vi "MainCLEO.vi"() -> ()   [LabVIEW 2013]
uses:
  Global.vi
  <vilib>/Utility/file.llb/Write To Spreadsheet File (string).vi
panel:
  in  "stop":bool
  in  "Measured values [mm]":i32(listbox)
  out "Standard deviation":dbl min=0.0 step=0.001 format="%.2f"
  out "Mean":dbl min=0.0 step=0.001 format="%.2f"
  out "Array":dbl[][](array[numeric])
  in  "Clear":bool
  out "String 3":string
  out "String 2":string
  in  "Radio Buttons":T1(radio)
  out "Delta average":dbl format="%#.4f"
  out "Delta right":dbl format="%#.4f"
  out "Delta left":dbl format="%#.4f"
  in  "Callibration event trigger":bool
  in  "Power monitor":bool
  out "Glass name":string
  in  "Load database":bool
  in  "Separator części dziesiętnych":enum32{". (kropka)", ", (przecinek)"}(radio)
  in  "Save to file":bool
  in  "Reset array":bool
  out "Results Array":string[][](array[string])
  out "Seria":i32(slide) max=20 scale=-1.0..3.0
  in  "Seryjny pomiar":bool
  out "Obecny pomiar":i32
  in  "Number of measurements":i32 min=1
  out "Bad average":bool
  out "Good average":bool
  out "Bad right":bool
  out "Good right":bool
  out "Measured thickness":dbl format="%.2f"
  in  "Wsp. komp.":dbl
  out "Bad left":bool
  out "Good left":bool
  in  "Tolerance +/-":dbl min=0.0 step=0.001 format="%.2f"
  in  "Target thickness":dbl min=0.0 step=0.001 format="%.2f"
  out "Lens thickness left":dbl format="%#.4f"
  out "Lens thickness right":dbl format="%#.4f"
  in  "Refractive index":dbl min=1.0
  in  "Pomiar":bool
  out "Peak position left":dbl
  out "Peak position right":dbl
  out "Peak coarse position":dbl
  out "Right peak":cluster{"Array":dbl[], "Array":dbl[]}(graph)
  out "Left peak":cluster{"Array":dbl[], "Array":dbl[]}(graph)
  out "Interferogram":cluster{"Array":dbl[], "Array":dbl[]}(graph)
  out "String":string
  out "Obecny proces":i32(slide) scale=0.0..9.0
  in  "Kalibracja":bool
  out "Karta do akwizycji danych":bool
  out "Układ pomiarowy":bool
  in  "Pomiar odchyłkowy":bool
  in  "Seryjny pomiar odchyłkowy":bool
  # "mm"
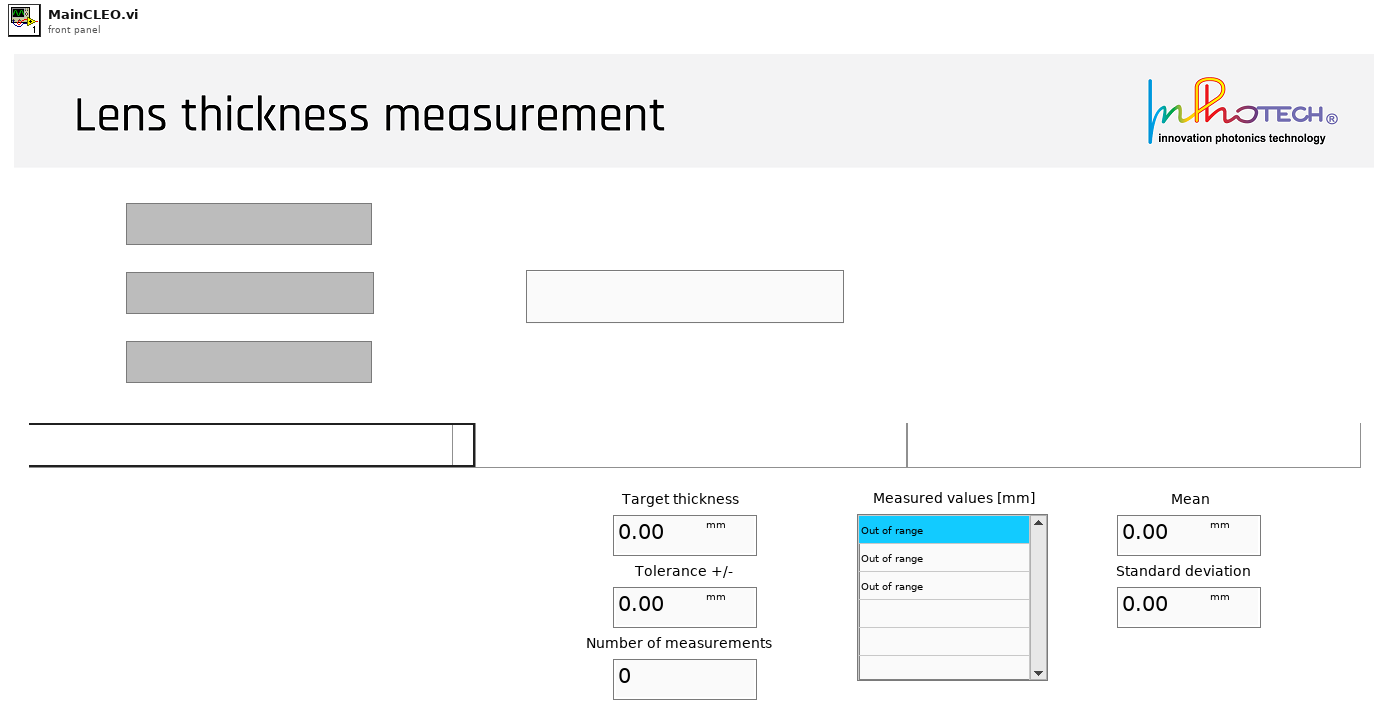
[diagram p1: front panel]
types:
  T1 = enum32{"Radio Selection 1", "Radio Selection 2", "Radio Selection 3"}
  T2 = cluster{"VISA resource name":refnum<visa-resource-name>, "Device name":string, "Controller address":i32, "error":errorcluster}
  T3 = enum8{"Enabled", "Disabled", "Disabled and Grayed Out"}
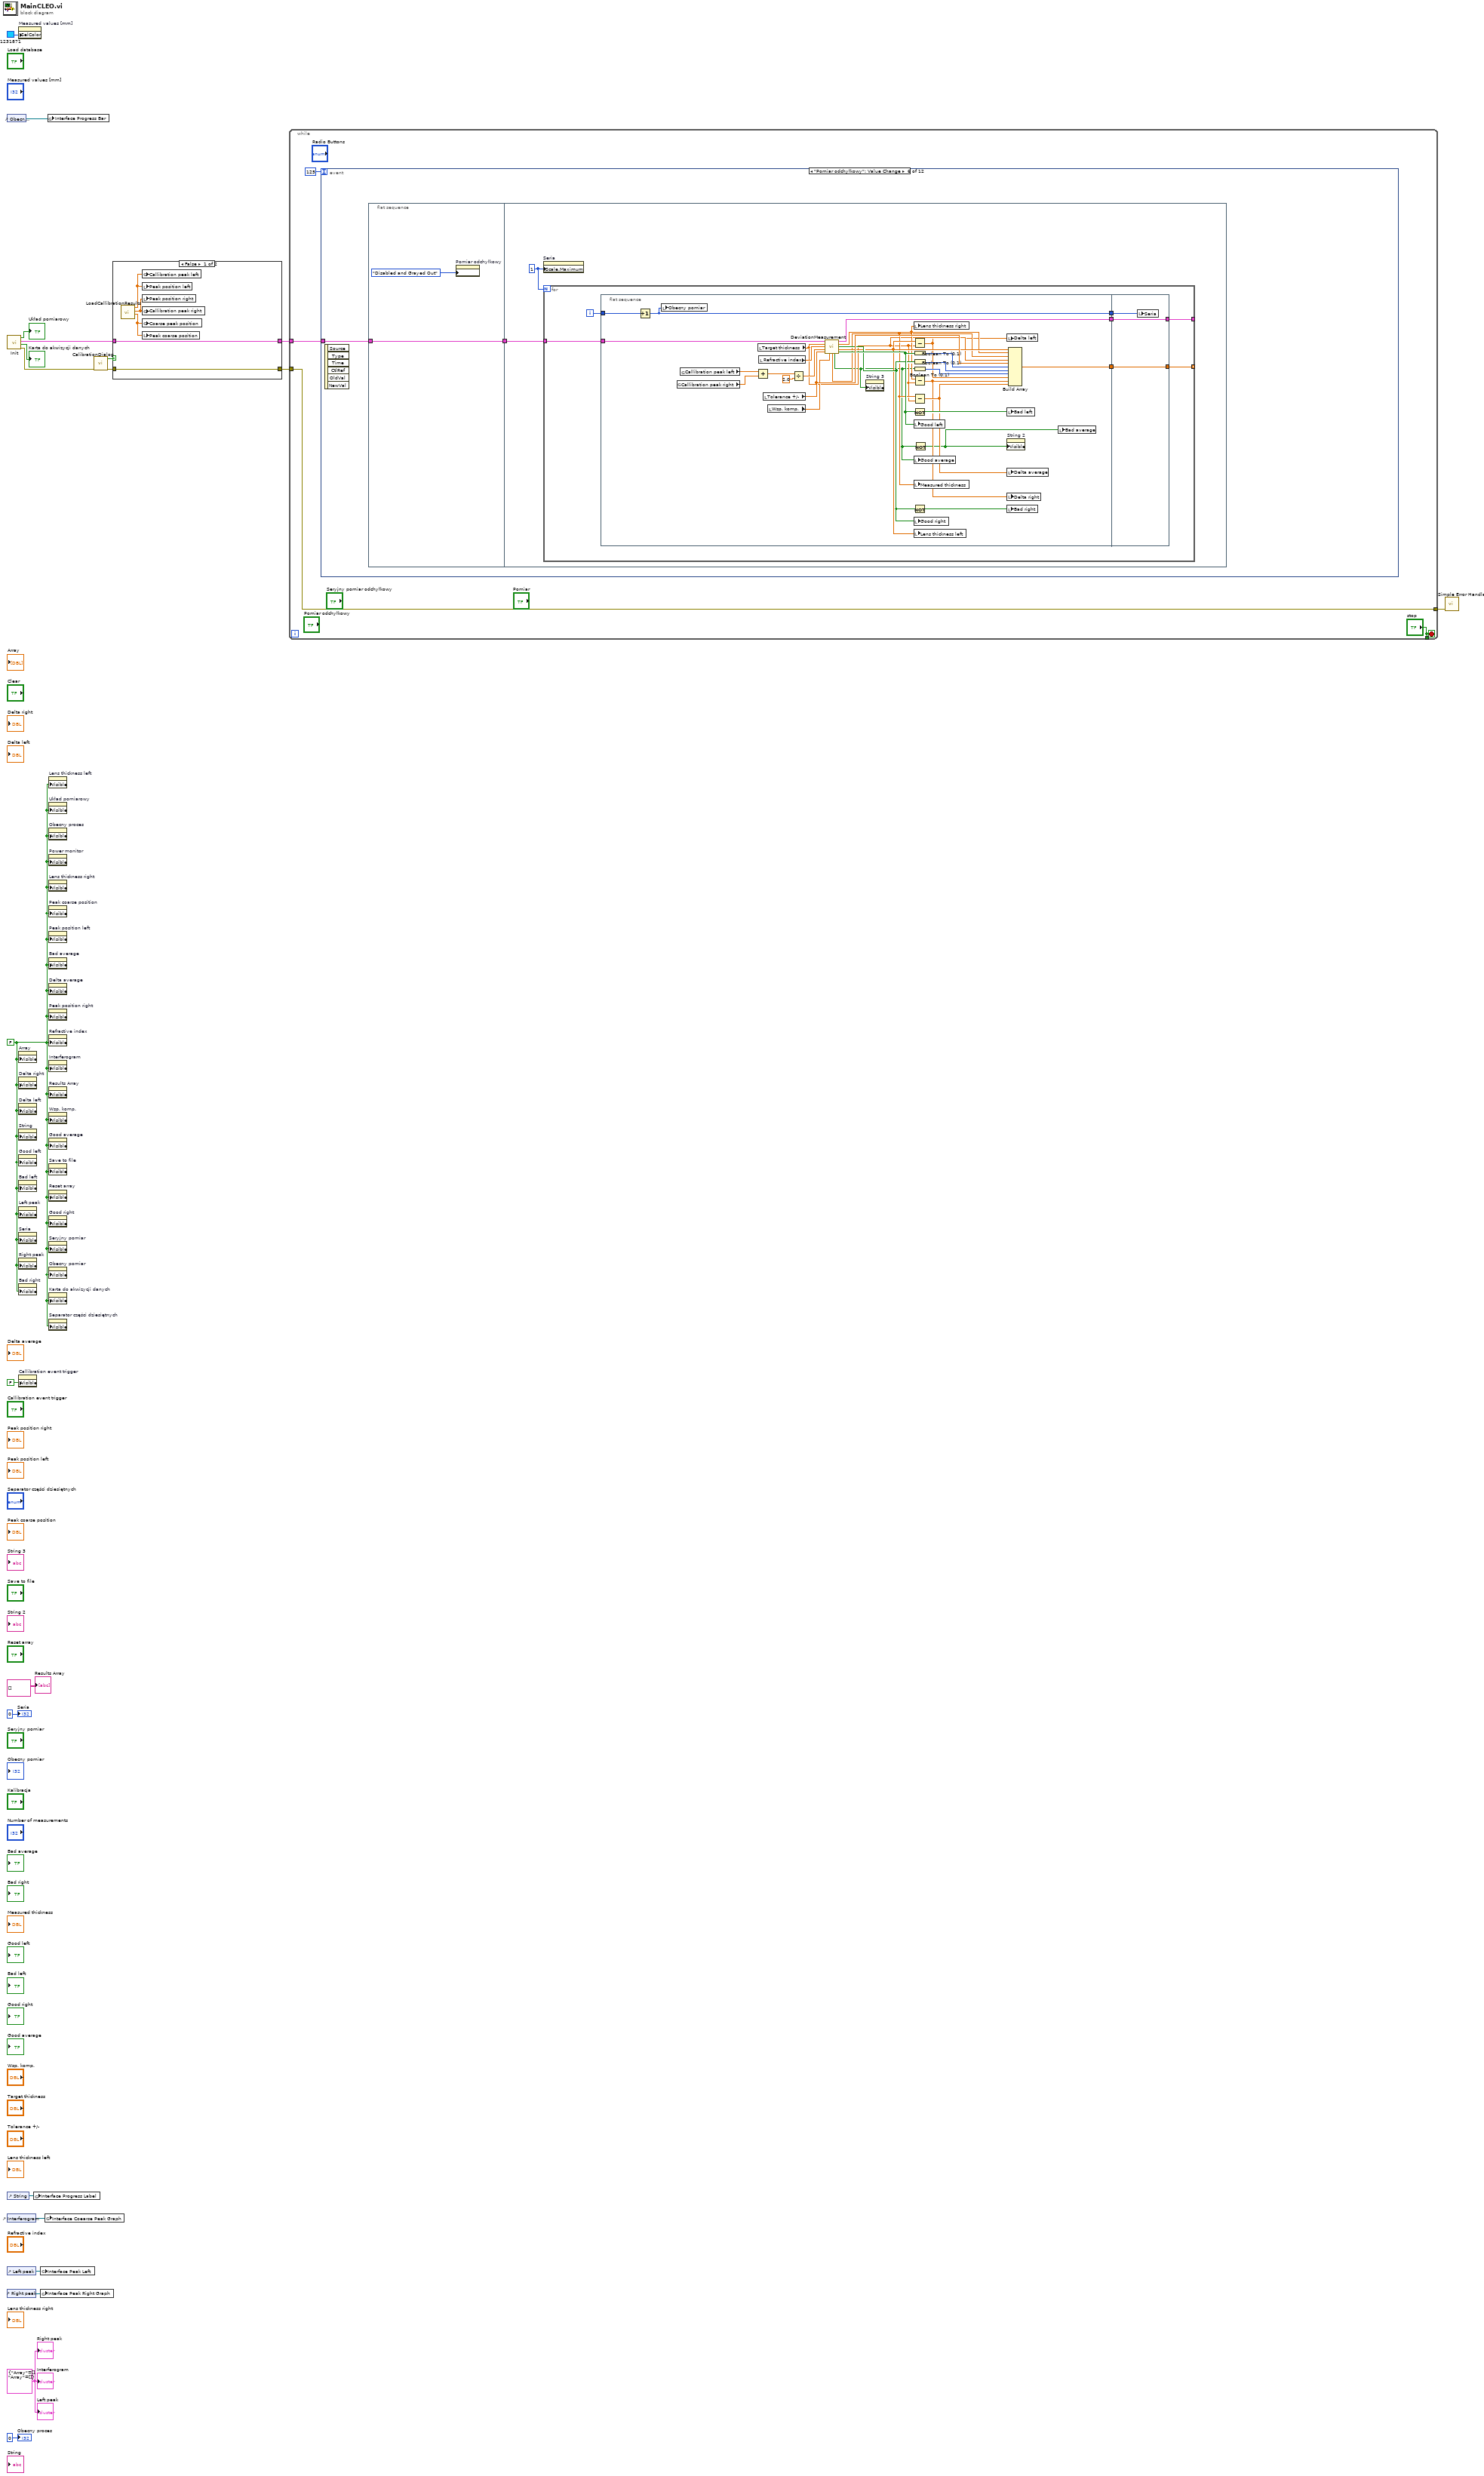
[diagram p0: block diagram]
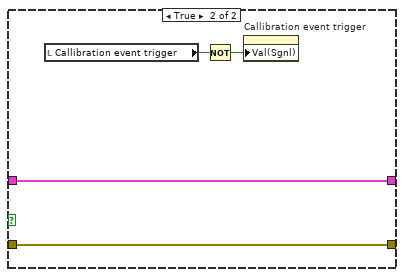
[diagram p2: hidden frame]
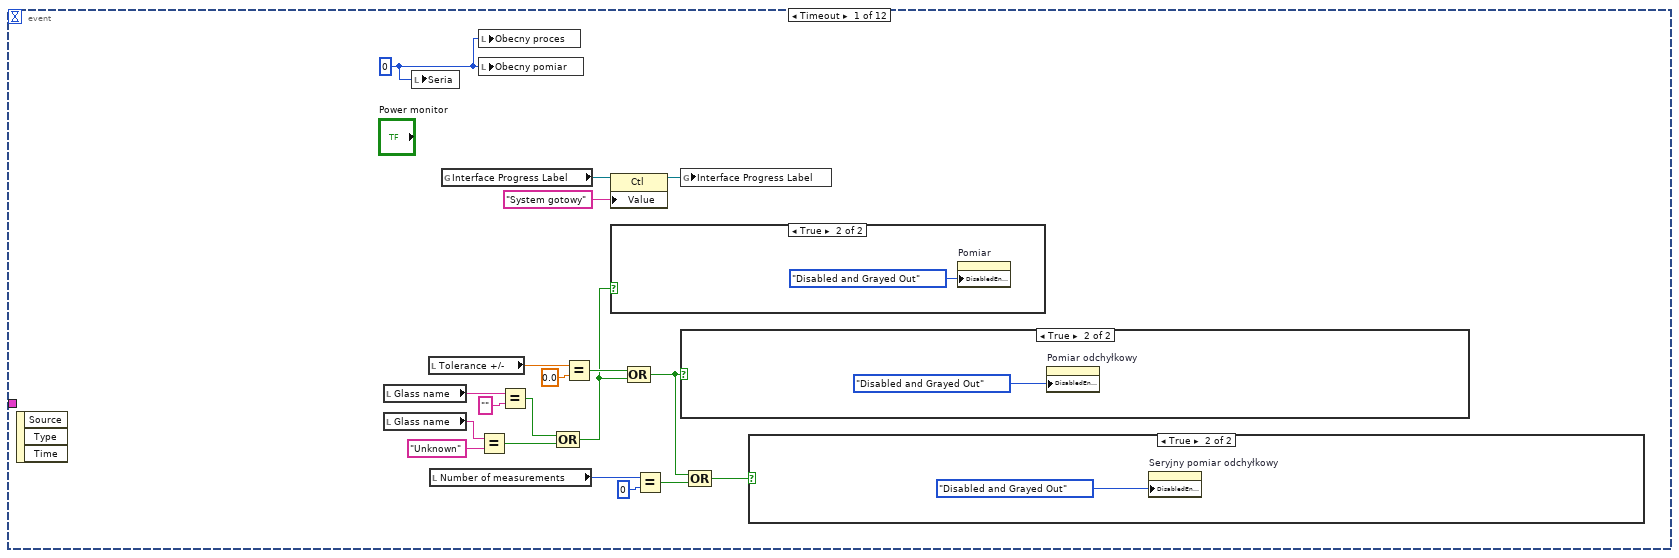
[diagram p3: hidden frame]
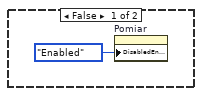
[diagram p4: hidden frame]
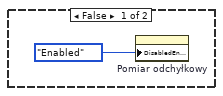
[diagram p5: hidden frame]
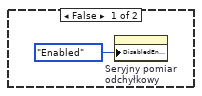
[diagram p6: hidden frame]
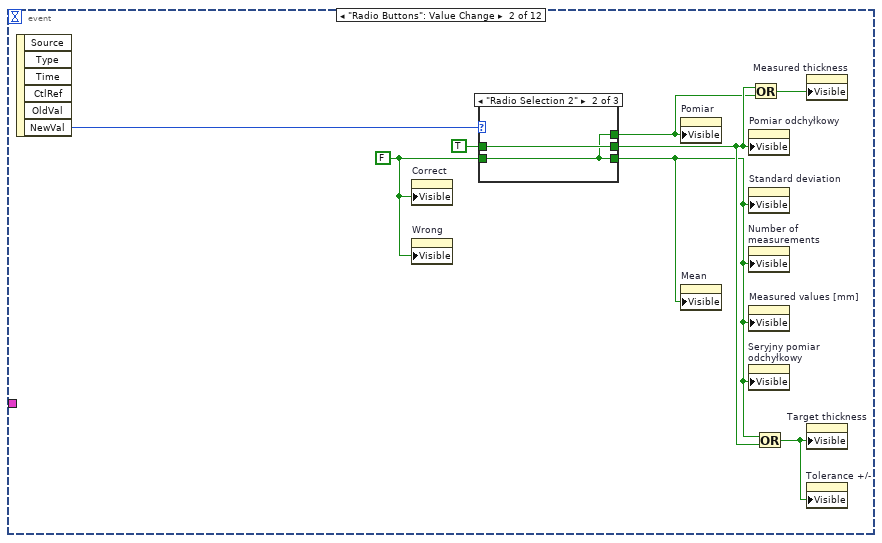
[diagram p7: hidden frame]
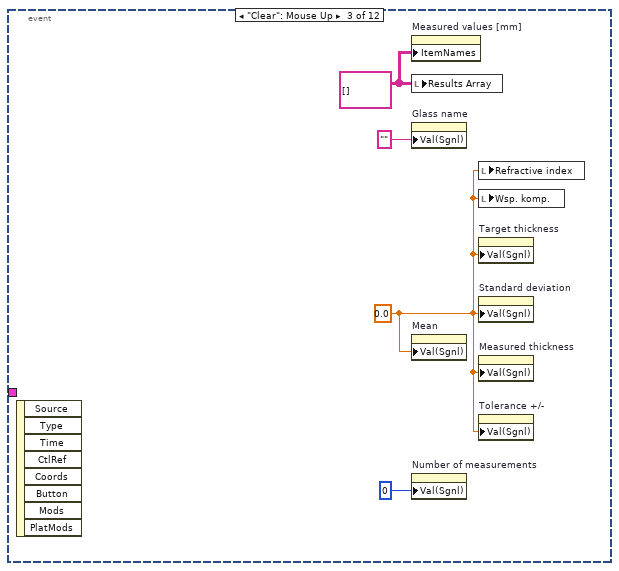
[diagram p10: hidden frame]
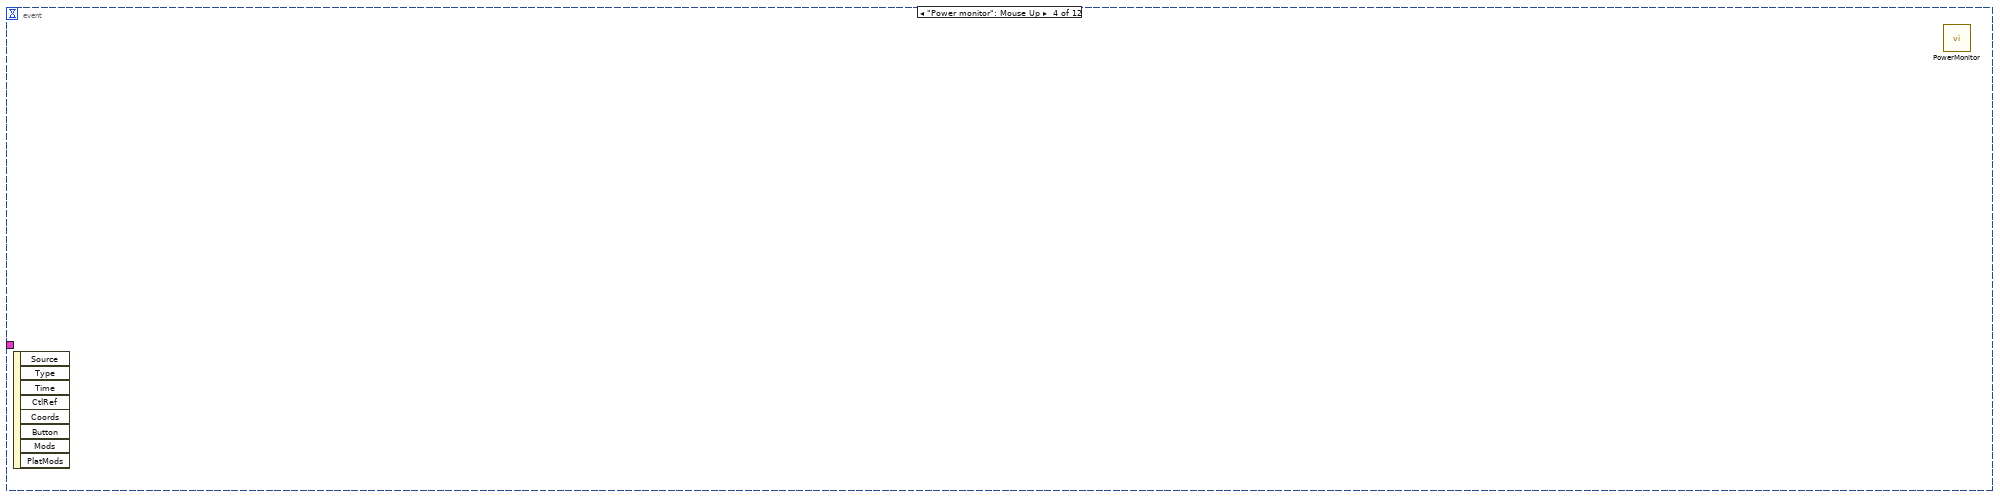
[diagram p11: hidden frame]
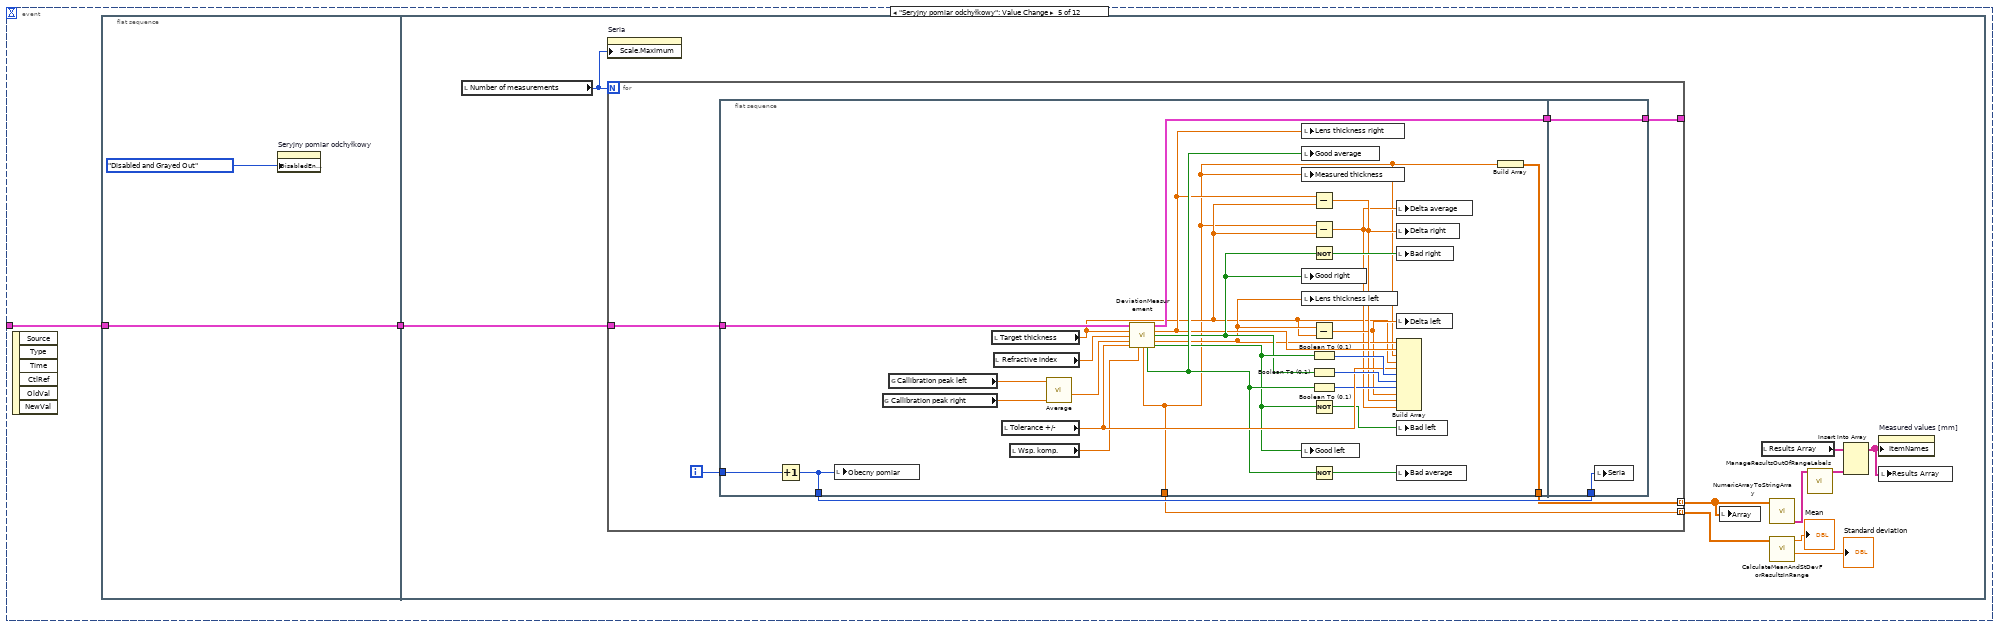
[diagram p12: hidden frame]
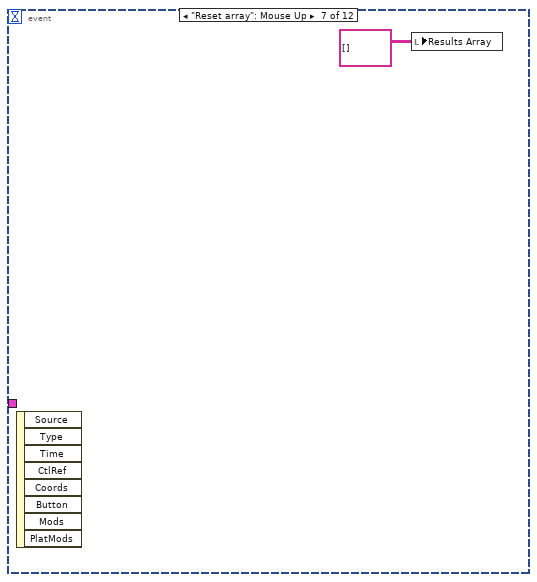
[diagram p13: hidden frame]
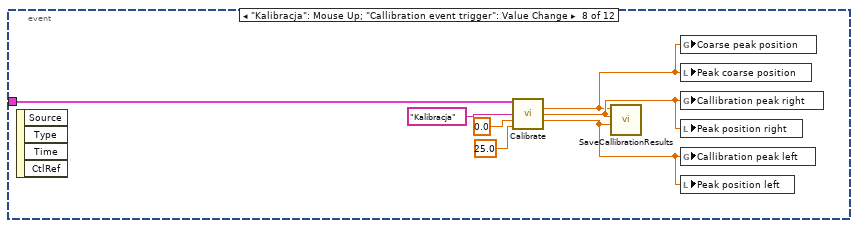
[diagram p14: hidden frame]
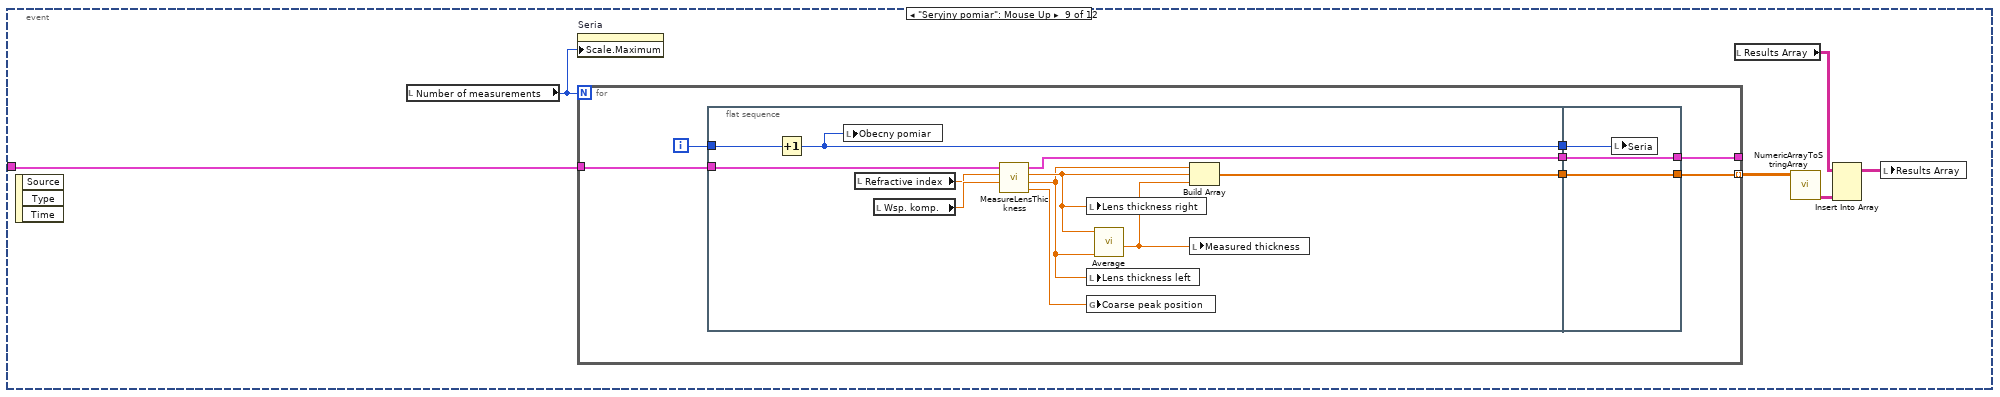
[diagram p15: hidden frame]
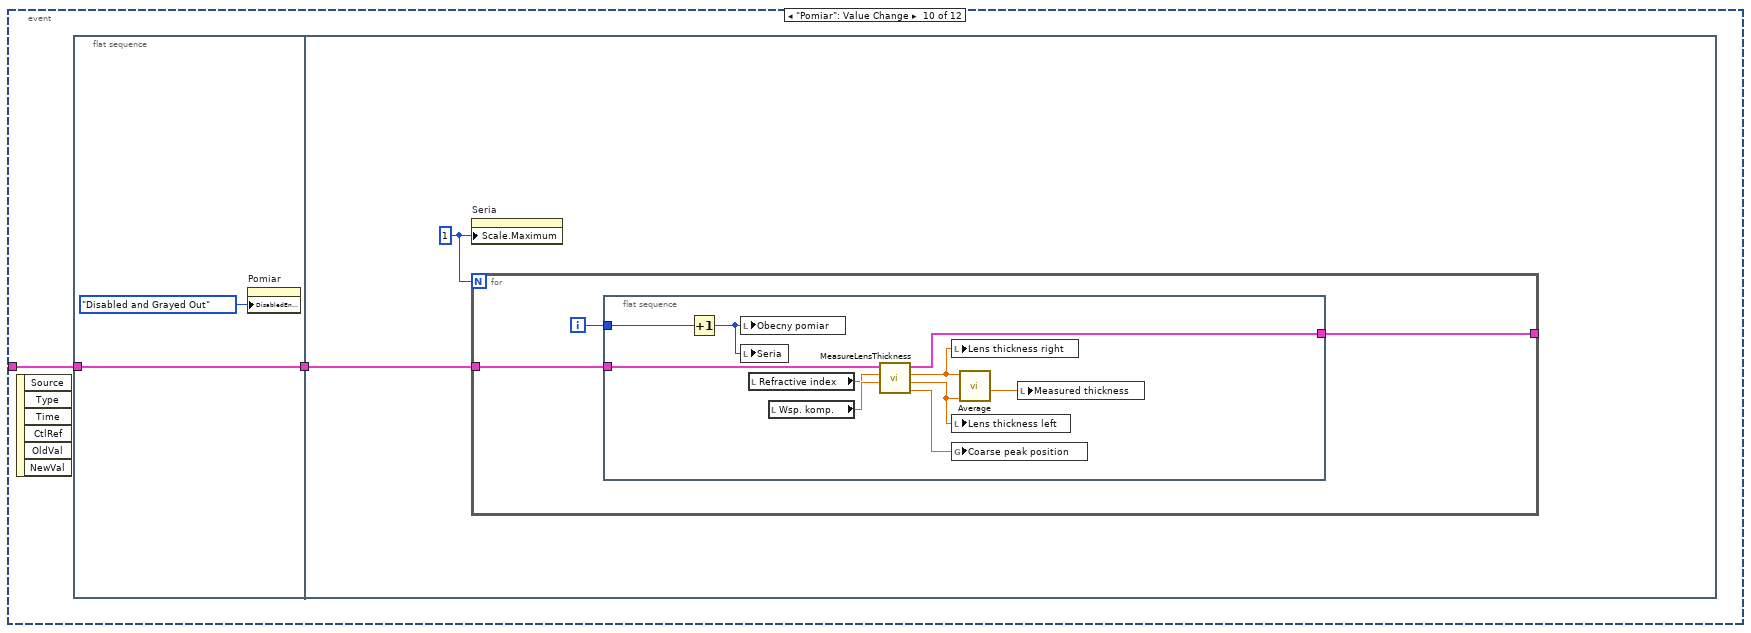
[diagram p16: hidden frame]
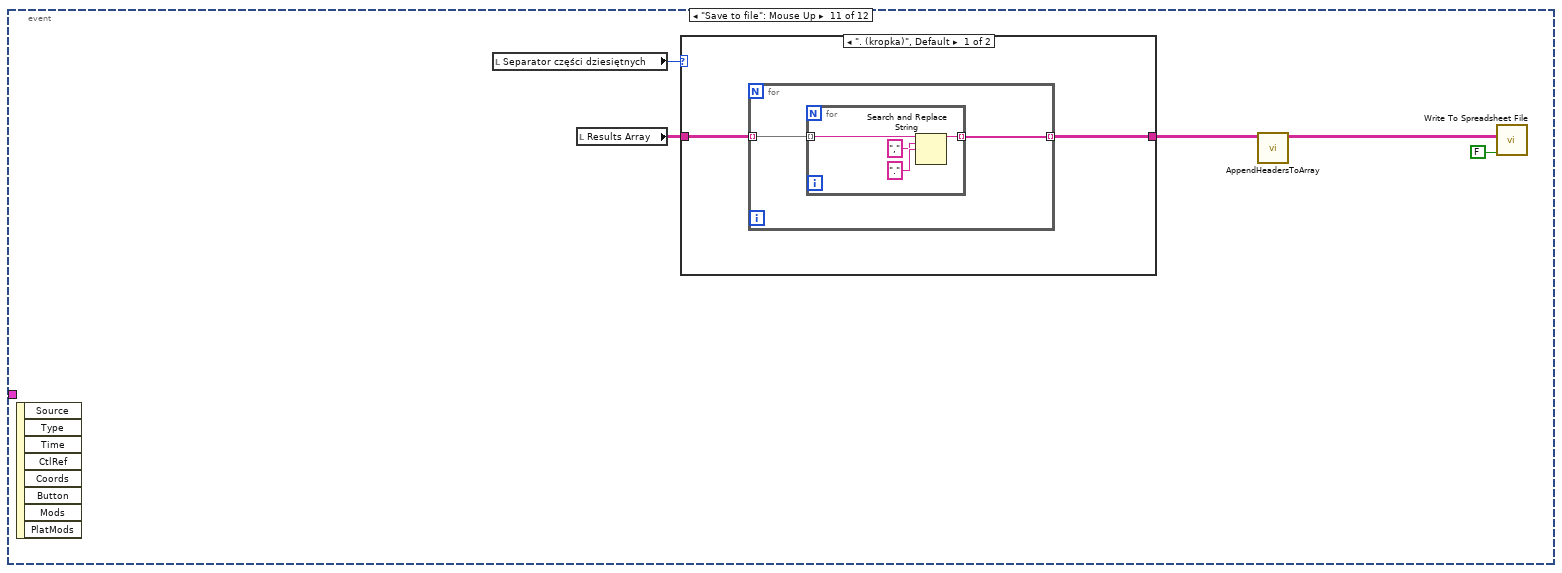
[diagram p17: hidden frame]
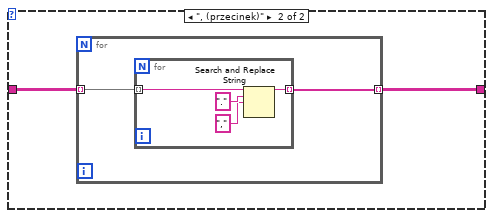
[diagram p18: hidden frame]
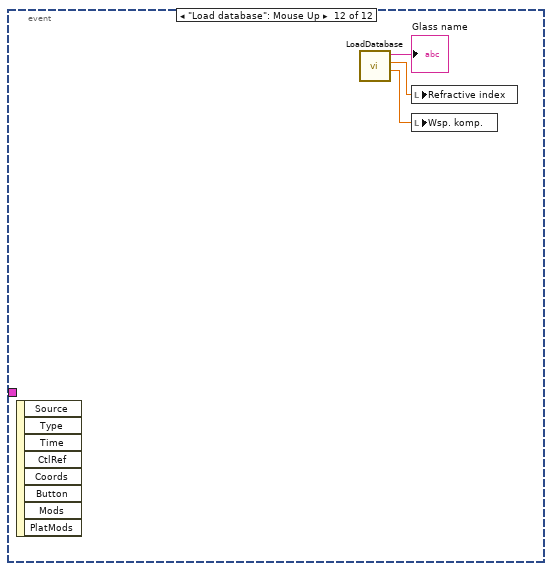
[diagram p19: hidden frame]
diagram:
  w1 = FALSE ("Visible")
  w3 = cluster{"Array":dbl[], "Array":dbl[]} {"Array"=[], "Array"=[]} ("Right peak")
  n1 = control-ref of="Obecny proces"() -> (w11:refnum<vi>)
  n2 = call "Init.vi"() -> ("error out"=w21:errorcluster, "DAQ"=→"Karta do akwizycji danych":bool, "Device Connection Cluster"=w14:T2, "Servo"=→"Układ pomiarowy":bool)  [unwired: 4 in]
  n3 = control-ref of="String"() -> (w10:refnum<vi>)
  n4 = control-ref of="Interferogram"() -> (w9:refnum<vi>)
  n5 = control-ref of="Left peak"() -> (w8:refnum<vi>)
  n6 = control-ref of="Right peak"() -> (w7:refnum<vi>)
  n7 = property on="Measured values [mm]" class="MCListbox (strict)"("SelColor"=u32 1231871) -> ()  [unwired: 2 in, 2 out]
  n8 = property on="Array" class="Arr (strict)"("Visible"=w1) -> ()  [unwired: 2 in, 2 out]
  n9 = property on="Delta right" class="DigNum (strict)"("Visible"=w1) -> ()  [unwired: 2 in, 2 out]
  n10 = property on="Delta left" class="DigNum (strict)"("Visible"=w1) -> ()  [unwired: 2 in, 2 out]
  n11 = property on="String" class="Str"("Visible"=w1) -> ()  [unwired: 2 in, 2 out]
  n12 = property on="Good left" class="Bool (strict)"("Visible"=w1) -> ()  [unwired: 2 in, 2 out]
  n13 = property on="Bad left" class="Bool (strict)"("Visible"=w1) -> ()  [unwired: 2 in, 2 out]
  n14 = property on="Left peak" class="XYGraph (strict)"("Visible"=w1) -> ()  [unwired: 2 in, 2 out]
  n15 = property on="Seria" class="Slide (strict)"("Visible"=w1) -> ()  [unwired: 2 in, 2 out]
  n16 = property on="Right peak" class="XYGraph (strict)"("Visible"=w1) -> ()  [unwired: 2 in, 2 out]
  n17 = property on="Bad right" class="Bool (strict)"("Visible"=w1) -> ()  [unwired: 2 in, 2 out]
  n18 = property on="Callibration event trigger" class="Bool (strict)"("Visible"=FALSE) -> ()  [unwired: 2 in, 2 out]
  n19 = global write "Global.vi" "Interface Progress Label"(w10) -> ()
  n20 = global write "Global.vi" "Interface Peak Left"(w8) -> ()
  n21 = global write "Global.vi" "Interface Peak Right Graph"(w7) -> ()
  n22 = global write "Global.vi" "Interface Coearse Peak Graph"(w9) -> ()
  n23 = global write "Global.vi" "Interface Progress Bar"(w11) -> ()
  n24 = property on="Lens thickness left" class="DigNum (strict)"("Visible"=w1) -> ()  [unwired: 2 in, 2 out]
  n25 = property on="Układ pomiarowy" class="Bool (strict)"("Visible"=w1) -> ()  [unwired: 2 in, 2 out]
  n26 = property on="Obecny proces" class="Slide (strict)"("Visible"=w1) -> ()  [unwired: 2 in, 2 out]
  n27 = property on="Power monitor" class="Bool"("Visible"=w1) -> ()  [unwired: 2 in, 2 out]
  n28 = property on="Lens thickness right" class="DigNum (strict)"("Visible"=w1) -> ()  [unwired: 2 in, 2 out]
  n29 = property on="Peak coarse position" class="DigNum (strict)"("Visible"=w1) -> ()  [unwired: 2 in, 2 out]
  n30 = property on="Peak position left" class="DigNum (strict)"("Visible"=w1) -> ()  [unwired: 2 in, 2 out]
  n31 = property on="Bad average" class="Bool (strict)"("Visible"=w1) -> ()  [unwired: 2 in, 2 out]
  n32 = property on="Delta average" class="DigNum (strict)"("Visible"=w1) -> ()  [unwired: 2 in, 2 out]
  n33 = property on="Peak position right" class="DigNum (strict)"("Visible"=w1) -> ()  [unwired: 2 in, 2 out]
  n34 = property on="Refractive index" class="DigNum (strict)"("Visible"=w1) -> ()  [unwired: 2 in, 2 out]
  n35 = property on="Interferogram" class="XYGraph (strict)"("Visible"=w1) -> ()  [unwired: 2 in, 2 out]
  n36 = property on="Results Array" class="Arr (strict)"("Visible"=w1) -> ()  [unwired: 2 in, 2 out]
  n37 = property on="Wsp. komp." class="DigNum (strict)"("Visible"=w1) -> ()  [unwired: 2 in, 2 out]
  n38 = property on="Good average" class="Bool (strict)"("Visible"=w1) -> ()  [unwired: 2 in, 2 out]
  n39 = property on="Save to file" class="Bool"("Visible"=w1) -> ()  [unwired: 2 in, 2 out]
  n40 = property on="Reset array" class="Bool"("Visible"=w1) -> ()  [unwired: 2 in, 2 out]
  n41 = property on="Good right" class="Bool (strict)"("Visible"=w1) -> ()  [unwired: 2 in, 2 out]
  n42 = property on="Seryjny pomiar" class="Bool (strict)"("Visible"=w1) -> ()  [unwired: 2 in, 2 out]
  n43 = property on="Obecny pomiar" class="DigNum (strict)"("Visible"=w1) -> ()  [unwired: 2 in, 2 out]
  n44 = property on="Karta do akwizycji danych" class="Bool (strict)"("Visible"=w1) -> ()  [unwired: 2 in, 2 out]
  n45 = property on="Separator części dziesiętnych" class="RadioBtnsControl (strict)"("Visible"=w1) -> ()  [unwired: 2 in, 2 out]
  n46 = call "CalibrationDialog.vi"("error in"=w21) -> ("error out"=w16:errorcluster, "Yes?"=w17:bool)  [unwired: 5 in]
  n47 = case shown="False" w17 {
    tunnel: w16 -> [w26 w30]
    tunnel: [w26 w30] -> w15
    tunnel: w14 -> [w25 w29]
    tunnel: [w25 w29] -> w13
    frame False {
      n48 = call "LoadCallibrationResults.vi"() -> ("Peak coarse"=w22:dbl, "Peak right"=w23:dbl, "Peak left"=w24:dbl)  [unwired: 9 in]
      n49 = global write "Global.vi" "Callibration peak left"(w24) -> ()
      n50 = local write "Peak position left"(w24) -> ()
      n51 = local write "Peak position right"(w23) -> ()
      n52 = global write "Global.vi" "Callibration peak right"(w23) -> ()
      n53 = global write "Global.vi" "Coarse peak position"(w22) -> ()
      n54 = local write "Peak coarse position"(w22) -> ()
    }
    frame True {
      n55 = local read "Callibration event trigger"() -> (w28:bool)
      n56 = Not(x=w28) -> (.not. x?=w27:bool)
      n57 = property on="Callibration event trigger" class="Bool (strict)"("Val(Sgnl)"=w27) -> ()  [unwired: 2 in, 2 out]
    }
  }
  n58 = while {
    tunnel: w15 -> [w34]
    tunnel: [w34] -> w18
    tunnel: w13 -> [w32]
    tunnel: ["stop"] -> _
    stop <- "stop" stop-if-true
    n59 = event shown="[5] \"Pomiar odchyłkowy\": Value Change" {
      selector: _ -> [_ _ _ _ _ _ _ _ _ _ _ _]
      dyn-events: _ -> [_ _ _ _ _ _ _ _ _ _ _ _]
      timeout: 125 -> [_ _ _ _ _ _ _ _ _ _ _ _]
      tunnel: w32 -> [_ _ _ _ w79 w129 _ w178 w186 w209 _ _]
      event Timeout {
        w50 = 0 ("Progress Bar")
        n60 = event-data() -> ()  [unwired: 1 in, 3 out]
        n61 = local read "Glass name"() -> (w47:string)
        n62 = local read "Glass name"() -> (w45:string)
        n63 = local write "Seria"(w50) -> ()
        n64 = local read "Tolerance +/-"() -> (w48:dbl)
        n65 = local read "Number of measurements"() -> (w42:i32)
        n66 = global read "Global.vi" "Interface Progress Label"() -> (w52:refnum<vi>)
        n67 = local write "Obecny proces"(w50) -> ()
        n68 = local write "Obecny pomiar"(w50) -> ()
        n69 = Equal?(x=w45, y="Unknown") -> (x = y?=w37:bool)
        n70 = Equal?(x=w47, y="") -> (x = y?=w36:bool)
        n71 = Compound Arithmetic op=OR(w36, w37) -> (w35:bool)
        n72 = Equal?(x=w48, y=0.0) -> (x = y?=w43:bool)
        n73 = property class="Ctl"(reference=w52, "Value"="System gotowy") -> (reference out=w51:refnum<vi>)  [unwired: 1 in, 1 out]
        n74 = case shown="True" w35 {
          frame False {
            n75 = property on="Pomiar" class="Bool (strict)"("DisabledEnum"=T3."Enabled" ("Disabled")) -> ()  [unwired: 2 in, 2 out]
          }
          frame True {
            n76 = property on="Pomiar" class="Bool (strict)"("DisabledEnum"=T3."Disabled and Grayed Out" ("Disabled")) -> ()  [unwired: 2 in, 2 out]
          }
        }
        n77 = Compound Arithmetic op=OR(w43, w35) -> (w40:bool)
        n78 = Equal?(x=w42, y=0) -> (x = y?=w39:bool)
        n79 = global write "Global.vi" "Interface Progress Label"(w51) -> ()
        n80 = case shown="True" w40 {
          frame False {
            n81 = property on="Pomiar odchyłkowy" class="Bool (strict)"("DisabledEnum"=T3."Enabled" ("Disabled")) -> ()  [unwired: 2 in, 2 out]
          }
          frame True {
            n82 = property on="Pomiar odchyłkowy" class="Bool (strict)"("DisabledEnum"=T3."Disabled and Grayed Out" ("Disabled")) -> ()  [unwired: 2 in, 2 out]
          }
        }
        n83 = Compound Arithmetic op=OR(w40, w39) -> (w38:bool)
        n84 = case shown="True" w38 {
          frame False {
            n85 = property on="Seryjny pomiar odchyłkowy" class="Bool (strict)"("DisabledEnum"=T3."Enabled" ("Disabled")) -> ()  [unwired: 2 in, 2 out]
          }
          frame True {
            n86 = property on="Seryjny pomiar odchyłkowy" class="Bool (strict)"("DisabledEnum"=T3."Disabled and Grayed Out" ("Disabled")) -> ()  [unwired: 2 in, 2 out]
          }
        }
      }
      event "Radio Buttons": Value Change {
        w64 = FALSE
        n87 = event-data() -> ("NewVal"=w67:T1)  [unwired: 1 in, 5 out]
        n88 = property on="Correct" class="Str"("Visible"=w64) -> ()  [unwired: 2 in, 2 out]
        n89 = property on="Wrong" class="Str"("Visible"=w64) -> ()  [unwired: 2 in, 2 out]
        n90 = case shown="\"Radio Selection 2\"" w67 {
          tunnel: TRUE -> [w69 w71 w73]
          tunnel: [w68 w70 w73] -> w60
          tunnel: w64 -> [w68 w70 w72]
          tunnel: [w68 w71 w72] -> w62
          tunnel: [w69 w70 w72] -> w61
          frame "Radio Selection 1", Default {
          }
          frame "Radio Selection 2" {
          }
          frame "Radio Selection 3" {
          }
        }
        n91 = property on="Pomiar" class="Bool (strict)"("Visible"=w61) -> ()  [unwired: 2 in, 2 out]
        n92 = property on="Mean" class="DigNum (strict)"("Visible"=w60) -> ()  [unwired: 2 in, 2 out]
        n93 = property on="Pomiar odchyłkowy" class="Bool (strict)"("Visible"=w62) -> ()  [unwired: 2 in, 2 out]
        n94 = property on="Standard deviation" class="DigNum (strict)"("Visible"=w60) -> ()  [unwired: 2 in, 2 out]
        n95 = property on="Number of measurements" class="DigNum (strict)"("Visible"=w60) -> ()  [unwired: 2 in, 2 out]
        n96 = property on="Measured values [mm]" class="MCListbox (strict)"("Visible"=w60) -> ()  [unwired: 2 in, 2 out]
        n97 = property on="Seryjny pomiar odchyłkowy" class="Bool (strict)"("Visible"=w60) -> ()  [unwired: 2 in, 2 out]
        n98 = Or(x=w62, y=w61) -> (x .or. y?=w63:bool)
        n99 = Or(x=w60, y=w62) -> (x .or. y?=w65:bool)
        n100 = property on="Measured thickness" class="DigNum (strict)"("Visible"=w63) -> ()  [unwired: 2 in, 2 out]
        n101 = property on="Target thickness" class="DigNum (strict)"("Visible"=w65) -> ()  [unwired: 2 in, 2 out]
        n102 = property on="Tolerance +/-" class="DigNum (strict)"("Visible"=w65) -> ()  [unwired: 2 in, 2 out]
      }
      event "Clear": Mouse Up {
        w75 = string[][] [] ("Item Names")
        w74 = 0.0 ("Value (Signaling)")
        n103 = event-data() -> ()  [unwired: 1 in, 8 out]
        n104 = property on="Measured values [mm]" class="MCListbox (strict)"("ItemNames"=w75) -> ()  [unwired: 2 in, 2 out]
        n105 = local write "Results Array"(w75) -> ()
        n106 = property on="Glass name" class="Str"("Val(Sgnl)"="") -> ()  [unwired: 2 in, 2 out]
        n107 = property on="Mean" class="DigNum (strict)"("Val(Sgnl)"=w74) -> ()  [unwired: 2 in, 2 out]
        n108 = property on="Number of measurements" class="DigNum (strict)"("Val(Sgnl)"=0) -> ()  [unwired: 2 in, 2 out]
        n109 = local write "Refractive index"(w74) -> ()
        n110 = local write "Wsp. komp."(w74) -> ()
        n111 = property on="Target thickness" class="DigNum (strict)"("Val(Sgnl)"=w74) -> ()  [unwired: 2 in, 2 out]
        n112 = property on="Standard deviation" class="DigNum (strict)"("Val(Sgnl)"=w74) -> ()  [unwired: 2 in, 2 out]
        n113 = property on="Measured thickness" class="DigNum (strict)"("Val(Sgnl)"=w74) -> ()  [unwired: 2 in, 2 out]
        n114 = property on="Tolerance +/-" class="DigNum (strict)"("Val(Sgnl)"=w74) -> ()  [unwired: 2 in, 2 out]
      }
      event "Power monitor": Mouse Up {
        n115 = event-data() -> ()  [unwired: 1 in, 8 out]
        n116 = call "PowerMonitor.vi"() -> ()  [unwired: 12 in]
      }
      event "Seryjny pomiar odchyłkowy": Value Change {
        n117 = event-data() -> ()  [unwired: 1 in, 6 out]
        n118 = flat-sequence {
          tunnel: w79 -> [w81]
          tunnel: [w81] -> w78
          tunnel: w78 -> [w91]
          frame #0 {
            n119 = property on="Seryjny pomiar odchyłkowy" class="Bool (strict)"("DisabledEnum"=T3."Disabled and Grayed Out" ("Disabled")) -> ()  [unwired: 2 in, 2 out]
          }
          frame #1 {
            n120 = local read "Number of measurements"() -> (w90:i32)
            n121 = property on="Seria" class="Slide (strict)"("Scale.Maximum"=w90) -> ()  [unwired: 2 in, 2 out]
            n122 = for {
              N: w90 -> [_]
              tunnel: w91 -> [w96]
              tunnel: [w93] -> w87 mode=indexing
              tunnel: [w95] -> _
              tunnel: [w92] -> w86 mode=indexing
              i -> [w98]
              n123 = flat-sequence {
                tunnel: w98 -> [w110]
                tunnel: [w101] -> w97
                tunnel: w96 -> [w109]
                tunnel: [w108] -> w94
                tunnel: [w100] -> w93
                tunnel: [w99] -> w92
                tunnel: w97 -> [w127]
                tunnel: [w126] -> w95
                tunnel: w94 -> [w126]
                frame #0 {
                  n124 = Increment(x=w110) -> (x+1=w101:i32)
                  n125 = local write "Obecny pomiar"(w101) -> ()
                  n126 = global read "Global.vi" "Callibration peak right"() -> (w124:dbl)
                  n127 = global read "Global.vi" "Callibration peak left"() -> (w123:dbl)
                  n128 = local read "Target thickness"() -> (w102:dbl)
                  n129 = local read "Refractive index"() -> (w111:dbl)
                  n130 = local read "Tolerance +/-"() -> (w120:dbl)
                  n131 = local read "Wsp. komp."() -> (w114:dbl)
                  n132 = call "Average.vi"("y"=w124, "x"=w123) -> ("Average"=w125:dbl)  [unwired: 9 in]
                  n133 = call "DeviationMeasurement.vi"("Connection Cluster in"=w109, "Wanted thickness"=w102, "Refractive Index"=w111, "Peak position"=w125, "Thickness range"=w120, "Compensation factor"=w114) -> ("Connection Cluster out"=w108:T2, "Lens thickness right"=w107:dbl, "Thickness right in range?"=w116:bool, "Lens thickness left"=w105:dbl, "Lens thickness average"=w99:dbl, "Lens thickness in range? average"=w118:bool, "Thickness left in range?"=w117:bool)  [unwired: 3 in]
                  n134 = local write "Lens thickness right"(w107) -> ()
                  n135 = local write "Good average"(w118) -> ()
                  n136 = local write "Measured thickness"(w99) -> ()
                  n137 = local write "Good right"(w116) -> ()
                  n138 = local write "Lens thickness left"(w105) -> ()
                  n139 = local write "Good left"(w117) -> ()
                  n140 = Subtract(x=w107, y=w102) -> (x-y=w106:dbl)
                  n141 = Subtract(x=w99, y=w102) -> (x-y=w103:dbl)
                  n142 = Not(x=w116) -> (.not. x?=w112:bool)
                  n143 = Subtract(x=w105, y=w102) -> (x-y=w104:dbl)
                  n144 = Boolean To (0,1)(Boolean=w117) -> (0, 1=w121:i16)
                  n145 = Boolean To (0,1)(Boolean=w116) -> (0, 1=w122:i16)
                  n146 = Boolean To (0,1)(Boolean=w118) -> (0, 1=w119:i16)
                  n147 = Not(x=w117) -> (.not. x?=w113:bool)
                  n148 = Not(x=w118) -> (.not. x?=w115:bool)
                  n149 = local write "Delta average"(w103) -> ()
                  n150 = local write "Delta right"(w106) -> ()
                  n151 = local write "Bad right"(w112) -> ()
                  n152 = local write "Delta left"(w104) -> ()
                  n153 = Build Array(w105, w107, w99, w102, w120, w121, w122, w119, w104, w106, w103) -> ()  [unwired: 1 out]
                  n154 = local write "Bad left"(w113) -> ()
                  n155 = local write "Bad average"(w115) -> ()
                  n156 = Build Array(w99) -> (w100:dbl[])
                }
                frame #1 {
                  n157 = local write "Seria"(w127) -> ()
                }
              }
            }
            n158 = local write "Array"(w87) -> ()
            n159 = local read "Results Array"() -> (w89:string[][])
            n160 = call "NumericArrayToStringArray.vi"("Array"=w87) -> ("Array 2"=w83:string[][])  [unwired: 10 in]
            n161 = call "CalculateMeanAndStDevForResultsInRange.vi"("X"=w86) -> ("standard deviation"=→"Standard deviation":dbl, "mean"=→"Mean":dbl)  [unwired: 9 in]
            n162 = call "ManageResultsOutOfRangeLabels.vi"("Input Array"=w83) -> ("Output Array"=w82:string[][])  [unwired: 10 in]
            n163 = Insert Into Array(array=w89, new element=w82) -> (w88:string[][])  [unwired: 2 in]
            n164 = property on="Measured values [mm]" class="MCListbox (strict)"("ItemNames"=w88) -> ()  [unwired: 2 in, 2 out]
            n165 = local write "Results Array"(w88) -> ()
          }
        }
      }
      event "Pomiar odchyłkowy": Value Change {
        n166 = event-data() -> ()  [unwired: 1 in, 6 out]
        n167 = flat-sequence {
          tunnel: w129 -> [w131]
          tunnel: [w131] -> w128
          tunnel: w128 -> [w133]
          frame #0 {
            n168 = property on="Pomiar odchyłkowy" class="Bool (strict)"("DisabledEnum"=T3."Disabled and Grayed Out" ("Disabled")) -> ()  [unwired: 2 in, 2 out]
          }
          frame #1 {
            w132 = 1
            n169 = property on="Seria" class="Slide (strict)"("Scale.Maximum"=w132) -> ()  [unwired: 2 in, 2 out]
            n170 = for {
              N: w132 -> [_]
              tunnel: w133 -> [w136]
              tunnel: [w140] -> _ mode=indexing
              tunnel: [w134] -> _
              i -> [w139]
              n171 = flat-sequence {
                tunnel: w139 -> [w153]
                tunnel: [w154] -> w138
                tunnel: [w152] -> w137
                tunnel: w136 -> [w151]
                tunnel: [w150] -> w135
                tunnel: [w172] -> w140
                tunnel: w138 -> [w172]
                tunnel: w137 -> [w171]
                tunnel: [w170] -> w134
                tunnel: w135 -> [w170]
                frame #0 {
                  n172 = Increment(x=w153) -> (x+1=w152:i32)
                  n173 = local write "Obecny pomiar"(w152) -> ()
                  n174 = global read "Global.vi" "Callibration peak right"() -> (w157:dbl)
                  n175 = global read "Global.vi" "Callibration peak left"() -> (w156:dbl)
                  n176 = Add(x=w156, y=w157) -> (x+y=w159:dbl)
                  n177 = local read "Target thickness"() -> (w146:dbl)
                  n178 = local read "Refractive index"() -> (w155:dbl)
                  n179 = local read "Tolerance +/-"() -> (w167:dbl)
                  n180 = local read "Wsp. komp."() -> (w163:dbl)
                  n181 = Divide(x=w159, y=2.0) -> (x/y=w160:dbl)
                  n182 = call "DeviationMeasurement.vi"("Connection Cluster in"=w151, "Wanted thickness"=w146, "Refractive Index"=w155, "Peak position"=w160, "Thickness range"=w167, "Compensation factor"=w163) -> ("Connection Cluster out"=w150:T2, "Lens thickness right"=w148:dbl, "Thickness right in range?"=w164:bool, "Lens thickness left"=w149:dbl, "Lens thickness average"=w147:dbl, "Lens thickness in range? average"=w141:bool, "Thickness left in range?"=w165:bool)  [unwired: 3 in]
                  n183 = property on="String 3" class="Str"("Visible"=w141) -> ()  [unwired: 2 in, 2 out]
                  n184 = Subtract(x=w149, y=w146) -> (x-y=w145:dbl)
                  n185 = Boolean To (0,1)(Boolean=w165) -> (0, 1=w168:i16)
                  n186 = Boolean To (0,1)(Boolean=w164) -> (0, 1=w169:i16)
                  n187 = Boolean To (0,1)(Boolean=w141) -> (0, 1=w166:i16)
                  n188 = Subtract(x=w148, y=w146) -> (x-y=w143:dbl)
                  n189 = Subtract(x=w147, y=w146) -> (x-y=w144:dbl)
                  n190 = Not(x=w165) -> (.not. x?=w162:bool)
                  n191 = Not(x=w164) -> (.not. x?=w161:bool)
                  n192 = local write "Lens thickness right"(w148) -> ()
                  n193 = local write "Good left"(w165) -> ()
                  n194 = Not(x=w141) -> (.not. x?=w142:bool)
                  n195 = local write "Good average"(w141) -> ()
                  n196 = local write "Measured thickness"(w147) -> ()
                  n197 = local write "Good right"(w164) -> ()
                  n198 = local write "Lens thickness left"(w149) -> ()
                  n199 = local write "Delta left"(w145) -> ()
                  n200 = local write "Bad left"(w162) -> ()
                  n201 = property on="String 2" class="Str"("Visible"=w142) -> ()  [unwired: 2 in, 2 out]
                  n202 = local write "Delta average"(w144) -> ()
                  n203 = local write "Delta right"(w143) -> ()
                  n204 = local write "Bad right"(w161) -> ()
                  n205 = Build Array(w149, w148, w147, w146, w167, w168, w169, w166, w145, w143, w144) -> (w154:dbl[])
                  n206 = local write "Bad average"(w142) -> ()
                }
                frame #1 {
                  n207 = local write "Seria"(w171) -> ()
                }
              }
            }
          }
        }
      }
      event "Reset array": Mouse Up {
        n208 = event-data() -> ()  [unwired: 1 in, 8 out]
        n209 = local write "Results Array"(string[][] [] ("Array 2")) -> ()
      }
      event "Kalibracja": Mouse Up; "Callibration event trigger": Value Change {
        n210 = event-data() -> ()  [unwired: 1 in, 4 out]
        n211 = call "Calibrate.vi"("Connection Cluster in"=w178, "String"="Kalibracja", "Start position"=0.0, "Target position"=25.0 ("Start position")) -> ("Peak position"=w174:dbl, "Peak (right)"=w176:dbl, "Peak (left)"=w175:dbl)  [unwired: 8 in, 1 out]
        n212 = call "SaveCallibrationResults.vi"("Peak (left)"=w175, "Peak (right)"=w176, "Peak position"=w174) -> ()  [unwired: 9 in]
        n213 = global write "Global.vi" "Coarse peak position"(w174) -> ()
        n214 = local write "Peak coarse position"(w174) -> ()
        n215 = global write "Global.vi" "Callibration peak right"(w176) -> ()
        n216 = local write "Peak position right"(w176) -> ()
        n217 = global write "Global.vi" "Callibration peak left"(w175) -> ()
        n218 = local write "Peak position left"(w175) -> ()
      }
      event "Seryjny pomiar": Mouse Up {
        n219 = event-data() -> ()  [unwired: 1 in, 3 out]
        n220 = local read "Number of measurements"() -> (w185:i32)
        n221 = property on="Seria" class="Slide (strict)"("Scale.Maximum"=w185) -> ()  [unwired: 2 in, 2 out]
        n222 = for {
          N: w185 -> [_]
          tunnel: w186 -> [w189]
          tunnel: [w192] -> w182 mode=indexing
          tunnel: [w187] -> _
          i -> [w193]
          n223 = flat-sequence {
            tunnel: w193 -> [w197]
            tunnel: [w198] -> w191
            tunnel: [w196] -> w190
            tunnel: w189 -> [w195]
            tunnel: [w194] -> w188
            tunnel: [w207] -> w192
            tunnel: w191 -> [w207]
            tunnel: w190 -> [w206]
            tunnel: [w205] -> w187
            tunnel: w188 -> [w205]
            frame #0 {
              n224 = Increment(x=w197) -> (x+1=w196:i32)
              n225 = local write "Obecny pomiar"(w196) -> ()
              n226 = local read "Refractive index"() -> (w199:dbl)
              n227 = local read "Wsp. komp."() -> (w201:dbl)
              n228 = call "MeasureLensThickness.vi"("Compensation factor"=w201, "Refractive index"=w199, "Connection Cluster in"=w195) -> ("Peak position"=w200:dbl, "thickness left"=w203:dbl, "thickness right"=w204:dbl, "Connection Cluster out"=w194:T2)  [unwired: 5 in]
              n229 = local write "Lens thickness right"(w204) -> ()
              n230 = local write "Lens thickness left"(w203) -> ()
              n231 = global write "Global.vi" "Coarse peak position"(w200) -> ()
              n232 = call "Average.vi"("y"=w203, "x"=w204) -> ("Average"=w202:dbl)  [unwired: 9 in]
              n233 = Build Array(w203, w204, w202) -> (w198:dbl[])
              n234 = local write "Measured thickness"(w202) -> ()
            }
            frame #1 {
              n235 = local write "Seria"(w206) -> ()
            }
          }
        }
        n236 = local read "Results Array"() -> (w184:string[][])
        n237 = call "NumericArrayToStringArray.vi"("Array"=w182) -> ("Array 2"=w181:string[][])  [unwired: 10 in]
        n238 = Insert Into Array(array=w184, new element=w181) -> (w183:string[][])  [unwired: 2 in]
        n239 = local write "Results Array"(w183) -> ()
      }
      event "Pomiar": Value Change {
        n240 = event-data() -> ()  [unwired: 1 in, 6 out]
        n241 = flat-sequence {
          tunnel: w209 -> [w211]
          tunnel: [w211] -> w208
          tunnel: w208 -> [w213]
          frame #0 {
            n242 = property on="Pomiar" class="Bool (strict)"("DisabledEnum"=T3."Disabled and Grayed Out" ("Disabled")) -> ()  [unwired: 2 in, 2 out]
          }
          frame #1 {
            w212 = 1
            n243 = property on="Seria" class="Slide (strict)"("Scale.Maximum"=w212) -> ()  [unwired: 2 in, 2 out]
            n244 = for {
              N: w212 -> [_]
              tunnel: w213 -> [w215]
              tunnel: [w214] -> _
              i -> [w216]
              n245 = flat-sequence {
                tunnel: w216 -> [w219]
                tunnel: w215 -> [w218]
                tunnel: [w217] -> w214
                frame #0 {
                  n246 = Increment(x=w219) -> (x+1=w223:i32)
                  n247 = local write "Obecny pomiar"(w223) -> ()
                  n248 = local write "Seria"(w223) -> ()
                  n249 = local read "Refractive index"() -> (w220:dbl)
                  n250 = local read "Wsp. komp."() -> (w222:dbl)
                  n251 = call "MeasureLensThickness.vi"("Compensation factor"=w222, "Refractive index"=w220, "Connection Cluster in"=w218) -> ("Peak position"=w221:dbl, "thickness left"=w225:dbl, "thickness right"=w226:dbl, "Connection Cluster out"=w217:T2)  [unwired: 5 in]
                  n252 = local write "Lens thickness right"(w226) -> ()
                  n253 = local write "Lens thickness left"(w225) -> ()
                  n254 = global write "Global.vi" "Coarse peak position"(w221) -> ()
                  n255 = call "Average.vi"("y"=w225, "x"=w226) -> ("Average"=w224:dbl)  [unwired: 9 in]
                  n256 = local write "Measured thickness"(w224) -> ()
                }
              }
            }
          }
        }
      }
      event "Save to file": Mouse Up {
        n257 = event-data() -> ()  [unwired: 1 in, 8 out]
        n258 = local read "Separator części dziesiętnych"() -> (w230:enum32{". (kropka)", ", (przecinek)"})
        n259 = local read "Results Array"() -> (w229:string[][])
        n260 = case shown="\". (kropka)\", Default" w230 {
          tunnel: w229 -> [w233 w241]
          tunnel: [w232 w240] -> w228
          frame ". (kropka)", Default {
            n261 = for {
              tunnel: w233 -> [w235] mode=indexing
              tunnel: [w234] -> w232 mode=indexing
              n262 = for {
                tunnel: w235 -> [w237] mode=indexing
                tunnel: [w236] -> w234 mode=indexing
                n263 = Search and Replace String(input string=w237, search string=",", replace string="." ("replace string (\"\")")) -> (result string=w236:string)  [unwired: 5 in, 3 out]
              }
            }
          }
          frame ", (przecinek)" {
            n264 = for {
              tunnel: w241 -> [w243] mode=indexing
              tunnel: [w242] -> w240 mode=indexing
              n265 = for {
                tunnel: w243 -> [w247] mode=indexing
                tunnel: [w244] -> w242 mode=indexing
                n266 = Search and Replace String(input string=w247, search string=".", replace string="," ("replace string (\"\")")) -> (result string=w244:string)  [unwired: 5 in, 3 out]
              }
            }
          }
        }
        n267 = call "AppendHeadersToArray.vi"("Array"=w228) -> ("output array"=w227:string[][])  [unwired: 10 in]
        n268 = call-poly <vilib>:"Write To Spreadsheet File.vi"("append to file? (new file:F)"=FALSE, "2D data"=w227) -> ()  [unwired: 6 in, 1 out]
      }
      event "Load database": Mouse Up {
        n269 = event-data() -> ()  [unwired: 1 in, 8 out]
        n270 = call "LoadDatabase.vi"() -> ("Deispersion compenastion factor"=w248:dbl, "Refractive index"=w249:dbl, "Glass name"=→"Glass name":string)  [unwired: 9 in]
        n271 = local write "Refractive index"(w249) -> ()
        n272 = local write "Wsp. komp."(w248) -> ()
      }
    }
  }
  n273 = call <vilib>:"Simple Error Handler.vi"("error in (no error)"=w18) -> ()  [unwired: 4 in, 5 out]
  "Obecny proces" <- 0 ("Progress Bar")
  "Interferogram" <- w3
  "Left peak" <- w3
  "Right peak" <- w3
  "Seria" <- 0 ("Seria")
  "Results Array" <- string[][] [] ("Array 2")
